vi "speed_threshold.vi"(11 "SPEED IN":dbl) -> (3 "SPEED OUT":dbl)   [LabVIEW 2019]
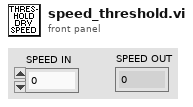
[diagram p1: front panel]
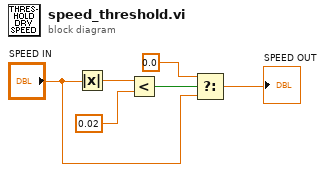
[diagram p0: block diagram]
diagram:
  n1 = Absolute Value(x="SPEED IN") -> (abs(x)=w6:dbl)
  n2 = Less?(x=w6, y=0.02) -> (x < y?=w3:bool)
  n3 = Select(t=0.0, s=w3, f="SPEED IN") -> (s? t:f=→"SPEED OUT":dbl)
